vi "get data interface information.vi"(10 "channel classification":T1, 11 "Temperature Chamber Model runtime in":refnum<class "Temperature Chamber Model runtime.lvclass">) -> (1 "valid?":bool, 2 "index cluster":variant, 3 "Temperature Chamber Model runtime out":refnum<class "Temperature Chamber Model runtime.lvclass">)   [LabVIEW 2013, in "Temperature Chamber Model runtime.lvclass"]
uses:
  Temperature Chamber Model runtime.lvclass
  <vilib>/NI/Tag Bus Module Framework/channel/channel classification.ctl
  parameter user data.ctl
  result user data.ctl
  <vilib>/NI/Tag Bus Module Framework/channel/TBM channel.lvclass
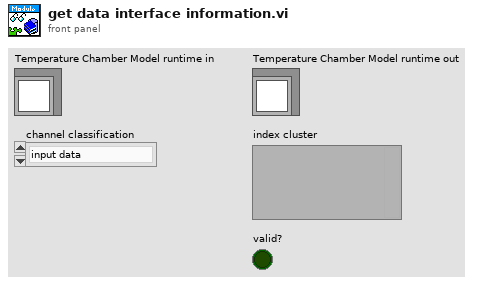
[diagram p1: front panel]
types:
  T1 = typedef "TBM channel.lvclass/channel classification.ctl" = enum16{"input data", "output data", "processing parameter", "processing result"}
  T2 = typedef "Temperature Chamber Model runtime.lvclass/parameter user data.ctl" = cluster{"Ambient Temperature":dbl, "Fan PWM":dbl, "Lamp PWM":dbl}
  T3 = typedef "Temperature Chamber Model runtime.lvclass/result user data.ctl" = cluster{"Thermocouple Reading":dbl}
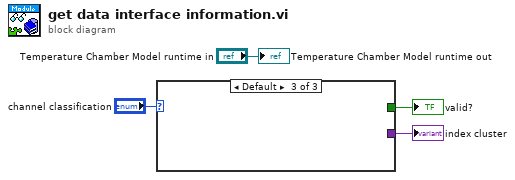
[diagram p0: block diagram]
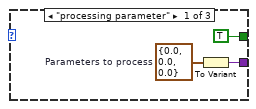
[diagram p2: hidden frame]
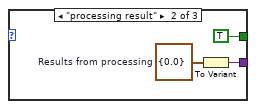
[diagram p3: hidden frame]
diagram:
  n1 = case shown="Default" "channel classification" {
    tunnel: [TRUE TRUE _] -> w2
    tunnel: [w7 w10 _] -> w1
    frame "processing parameter" {
      w5 = T2 {"Ambient Temperature"=0.0, "Fan PWM"=0.0, "Lamp PWM"=0.0}  # Parameters to process
      n2 = To Variant(anything=w5) -> (Variant=w7:variant)
    }
    frame "processing result" {
      w8 = T3 {"Thermocouple Reading"=0.0}  # Results from processing
      n3 = To Variant(anything=w8) -> (Variant=w10:variant)
    }
    frame Default {
    }
  }
  "valid?" <- w2
  "index cluster" <- w1
  "Temperature Chamber Model runtime out" <- "Temperature Chamber Model runtime in"
